vi "close.vi"(0 "object in":refnum<class "MBinteractive.lvclass">, 5 "error in (no error)":errorcluster) -> (14 "object out":refnum<class "MBinteractive.lvclass">, 19 "error out":errorcluster)   [LabVIEW 2016, in "MBinteractive.lvclass"]
uses:
  MBinteractive.lvclass
  MBinteractive.lvclass/MBinteractive.ctl
  <vilib>/NI/Modbus Library/API/Modbus API.lvclass
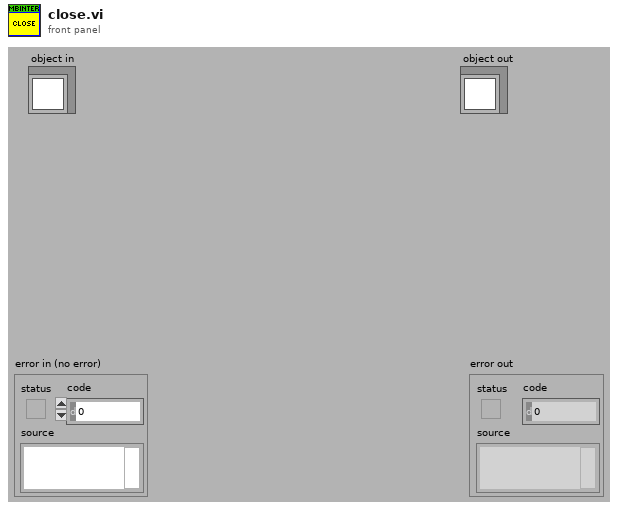
[diagram p1: front panel]
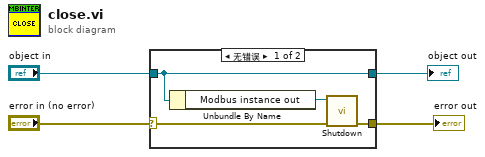
[diagram p0: block diagram]
diagram:
  n1 = case shown="无错误" "error in (no error)" {
    selector: "error in (no error)" -> [w8 w10]
    tunnel: [w6 w10] -> w3
    tunnel: [w5 w9] -> w1
    tunnel: "object in" -> [w5 w9]
    frame No Error {
      n2 = Unbundle By Name(w5) -> ("Modbus instance out"=w7:refnum<class "Modbus API.lvclass">)
      n3 = call-dynamic "Shutdown.vi"("error in"=w8, "Modbus instance in"=w7) -> ("error out"=w6:errorcluster)  [unwired: 9 in]
    }
    frame Error {
    }
  }
  "error out" <- w3
  "object out" <- w1
